vi "SiosIfmRawValue.vi"(1 "channel":i32, 2 "int32DeviceNumber":i32) -> (0 "rawValue":i64)   [LabVIEW 2009]
uses:
  siosifm.dll
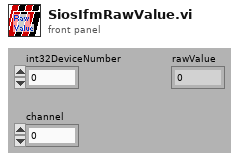
[diagram p1: front panel]
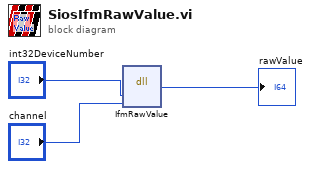
[diagram p0: block diagram]
diagram:
  n1 = dll-call lib="D:/Support/Labview/RE-10/SIOS_IfmDLL/siosifm.dll" fn="IfmRawValue"("deviceNumber"="int32DeviceNumber", "channel"="channel") -> ("rawValue"=→"rawValue":i64)  [unwired: 5 in, 2 out]
